vi "pH_monitor_calc.vi"(1 "Curent E Values":dbl[](array[numeric]), 2 "E0 Values":dbl[](array[numeric]), 3 "Cell Temp":dbl, 4 "Alkalinity Calculation Functions":T1) -> (0 "pH Values":dbl[](array[numeric]))   [LabVIEW 2010]
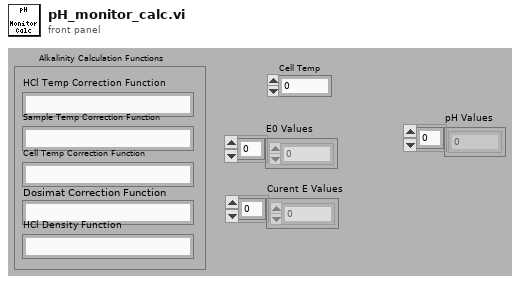
[diagram p1: front panel]
types:
  T1 = cluster{"HCl Temp Correction Function":string, "Sample Temp Correction Function":string, "Dosimat Correction Function":string, "Cell Temp Correction Function":string, "HCl Density Function":string}
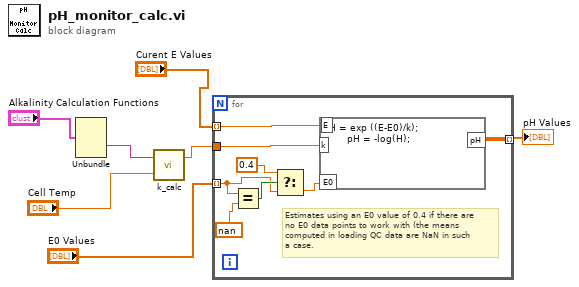
[diagram p0: block diagram]
diagram:
  n1 = Unbundle("Alkalinity Calculation Functions") -> ("Cell Temp Correction Function"=w6:string)  [unwired: 4 out]
  n2 = call "k_calc.vi"("Cell Temp"="Cell Temp", "Cell Temp Correction Formula"=w6) -> ("k"=w4:dbl)  [unwired: 1 out]
  n3 = for {
    tunnel: w4 -> [w15]
    tunnel: "Curent E Values" -> [w14] mode=indexing
    tunnel: "E0 Values" -> [w9] mode=indexing
    tunnel: [w13] -> w1 mode=indexing
    # "Estimates using an E0 value of 0.4 if there are\nno E0 data points to work with (the means\ncomputed in loading QC data are NaN in such\na case."
    n4 = Equal?(x=w9, y=nan) -> (x = y?=w10:bool)
    n5 = Select(t=0.4, s=w10, f=w9) -> (s? t:f=w12:dbl)
    n6 = formula code="H = exp ((E-E0)/k);\n      pH = -log(H);"("E0"=w12, "E"=w14, "k"=w15) -> ("pH"=w13:dbl)
  }
  "pH Values" <- w1
